vi "Determine if Running in Debug Mode.vi"(9 "App.Args":string[](array[string]), 10 "App.Kind":T1(ring), 11 "Launcher VI ref":refnum<vi>) -> (2 "Debug mode?":bool)   [LabVIEW 2024, in "Launcher Support.lvlib"]
doc: "The launcher VI is meant to be run as a headless launcher for the module main VI. The launcher VI can be used as a debugging tool.\n\nThis VI determines if the launcher VI is running as a debugger by parsing the command line arguments or checking if the VI is running in development mode and sets the Launcher VI properties accordingly.\n_____\nBased on DQMH Dev Tools: Project Template 7.1.0.1503."
uses:
  Launcher Support.lvlib
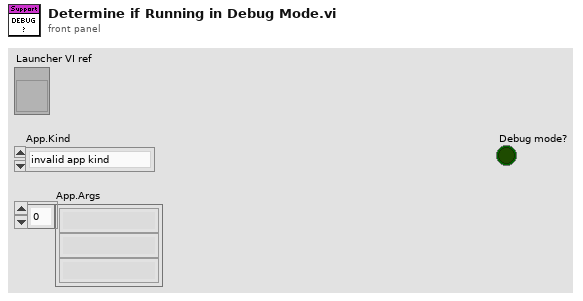
[diagram p1: front panel]
types:
  T1 = enum32{"invalid app kind", "Development System", "Run Time System", "Student Edition", "Embedded LabVIEW", "Evaluation", "Custom"}
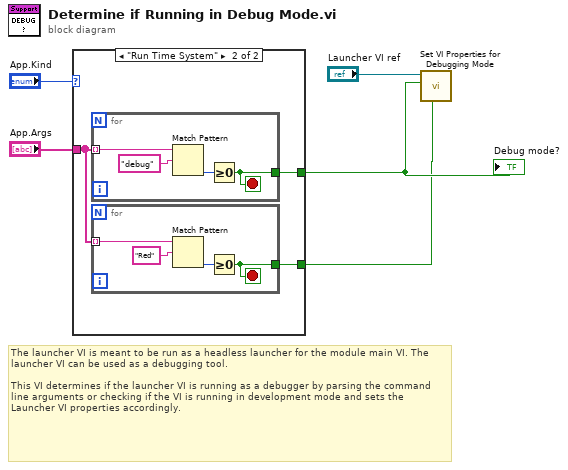
[diagram p0: block diagram]
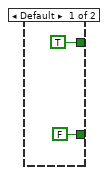
[diagram p2: hidden frame]
diagram:
  # "The launcher VI is meant to be run as a headless launcher for the module main VI. The launcher VI can be used as a debugging tool.\n\nThis VI determines if the launcher VI is running as a debugger by parsing the command line arguments or checking if the VI is running in development mode and sets the Launcher VI properties accordingly."
  n1 = case shown="\"Run Time System\"" "App.Kind" {
    tunnel: "App.Args" -> [_ w9]
    tunnel: [TRUE w10] -> w5
    tunnel: [FALSE w8] -> w1
    frame Default {
    }
    frame "Run Time System" {
      n2 = for {
        tunnel: w9 -> [w18] mode=indexing
        tunnel: [w15] -> w10
        stop <- w15 stop-if-true
        n3 = Match Pattern(string=w18, regular expression="debug") -> (offset past match=w16:i32)  [unwired: 1 in, 3 out]
        n4 = Greater Or Equal To 0?(x=w16) -> (x >= 0?=w15:bool)
      }
      n5 = for {
        tunnel: w9 -> [w14] mode=indexing
        tunnel: [w11] -> w8
        stop <- w11 stop-if-true
        n6 = Match Pattern(string=w14, regular expression="Red") -> (offset past match=w12:i32)  [unwired: 1 in, 3 out]
        n7 = Greater Or Equal To 0?(x=w12) -> (x >= 0?=w11:bool)
      }
    }
  }
  "Debug mode?" <- w5
  n8 = call "Set VI Properties for Debugging Mode.vi"("Red?"=w1, "Debug mode?"=w5, "Launcher VI ref"="Launcher VI ref") -> ()  [unwired: 7 in, 2 out]
